vi "myRIO_BRig_RT__Case_Exp_State_Cue1__v2.vi"(6 "input_LC":bool, 7 "I_lick":bool, 8 "input_LC_led":bool, 10 "input_state":T1, 11 "input_dataCurrent":u16[](array[numeric])) -> (0 "output_trigger_laser_led":bool, 2 "output_state":T1, 3 "output_dataCurrent":u16[](array[numeric]), 4 "output_trigger_laser":bool)   [LabVIEW 2014]
uses:
  myRIO_BRig_RT__Case_Exp_stateList.ctl
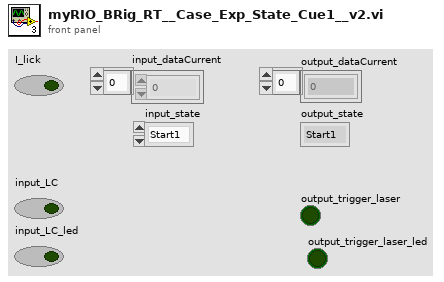
[diagram p1: front panel]
types:
  T1 = typedef "myRIO_BRig_RT__Case_Exp_stateList.ctl" = enum16{"Start1", "Start2", "Start3", "saveSettings1", "saveSettings2", "saveSettings3", "saveSettings4_LC_l1_ENL", "saveSettings4_LC_l2_ENL", "saveSettings5_LC_l1_Cue", "saveSettings5_LC_l2_Cue", "saveSettings6_LC_l1_Other", "SaveSettings6_LC_l2_Other", "setSettings_Audio", "setSettings_Laser", "initBlock_pre", "initBlock", "initBlock2", "initBlock_post", "initTrial_pre", "initTrial", "initTrial2", "initTrial3", "initTrial4", "initTrial_LC_ENL1", "initTrial_LC_Cue1", "initTrial_LC_Sel", "initTrial_post", "ENL1_pre", "ENL1", "ENL1_post", "ENL1Penalty_pre", "ENL1Penalty", "ENL2_pre", "ENL2", "ENL2Penalty_pre", "ENL2Penalty", "Cue1_pre", "Cue1", "Cue1_post", "Cue1Penalty_pre", "Cue1Penalty", "Cue2_pre", "Cue2", "Cue2Penalty_pre", "Cue2Penalty", "Selection_pre", "Selection", "Select_post", "SelectReward_pre", "SelectReward", "SelectRewardPost_pre", "SelectRewardPost", "SelectWrong_pre", "SelectWrong", "SelectWrong_post", "SelectTimeout_pre", "SelectTimeout", "SelectTimeout_post", "endTrial_pre", "endTrial1", "endTrial2", "endTrial3", "endTrial_post", "endBlock_pre", "endBlock", "endBlock_post", "endExp", "commConnect", "commUpload_pre", "commUpload_dataBlock", "commUpload_dataCurrent", "commUpload_dataExp", "commUpload_dataLC", "commUpload_dataTrial", "commUpload_post", "saveData_pre", "saveData_dataBlock", "saveData_dataCurrent", "saveData_dataExp", "saveData_dataLC", "saveData_dataTrial", "saveData_post", "empty_endBlock1", "empty_endBlock2", "empty_endTrial1", "empty_endTrial2", "empty_endTrial3", "empty_endTrial4", "empty_endTrial5", "dummyState", "dummyState_endBlock"}
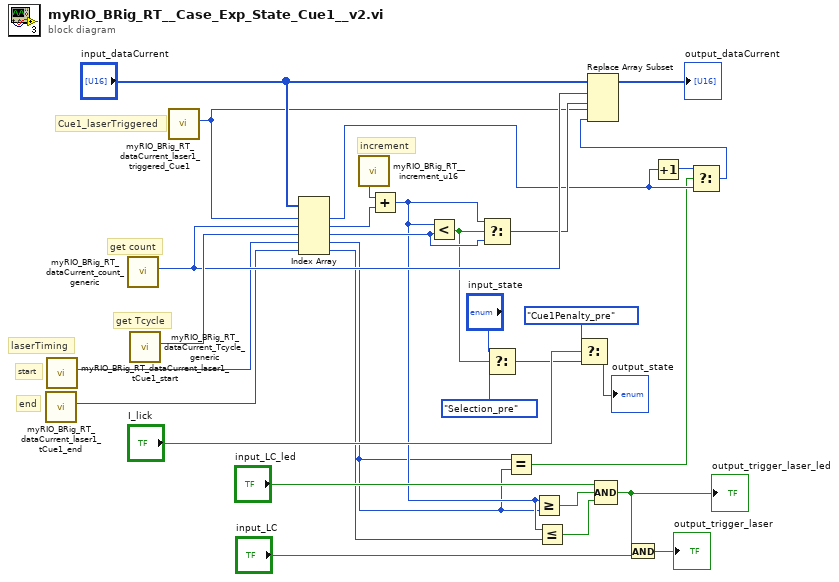
[diagram p0: block diagram]
diagram:
  # "Cue1_laserTriggered"
  # "end"
  # "start"
  # "laserTiming"
  # "increment"
  # "get Tcycle"
  # "get count"
  n1 = call "myRIO_BRig_RT_dataCurrent_laser1_tCue1_end.vi"() -> ("output_laser1_tCue1_end"=w9:i32)  [unwired: 11 in]
  n2 = call "myRIO_BRig_RT_dataCurrent_laser1_tCue1_start.vi"() -> ("output_laser1_tCue1_start"=w10:i32)  [unwired: 11 in]
  n3 = call "myRIO_BRig_RT_dataCurrent_count_generic.vi"() -> ("output_count_generic"=w28:i32)  [unwired: 11 in]
  n4 = call "myRIO_BRig_RT_dataCurrent_Tcycle_generic.vi"() -> ("output_Tcycle_generic"=w29:i32)  [unwired: 11 in]
  n5 = call "myRIO_BRig_RT_dataCurrent_laser1_triggered_Cue1.vi"() -> ("output_laser1_triggered_Cue1"=w8:i32)  [unwired: 11 in]
  n6 = Index Array(array="input_dataCurrent", index #1=w8, index #2=w28, index #3=w29, index #4=w10, index #5=w9) -> (element #1=w6:u16, element #2=w3:u16, element #3=w27:u16, element #4=w1:u16, element #5=w13:u16)
  n7 = call "myRIO_BRig_RT__increment_u16.vi"() -> ("output_increment__u16"=w22:u16)  [unwired: 11 in]
  n8 = Add(x=w22, y=w3) -> (x+y=w4:u16)
  n9 = Less?(x=w4, y=w27) -> (x < y?=w24:bool)
  n10 = Select(t=w4, s=w24, f=w27) -> (s? t:f=w26:u16)
  n11 = Select(t="input_state", s=w24, f=myRIO_BRig_RT__Case_Exp_stateList."Selection_pre" ("Enum")) -> (s? t:f=w23:T1)
  n12 = Equal?(x=w1, y=w1) -> (x = y?=w2:bool)
  n13 = Greater Or Equal?(x=w4, y=w1) -> (x >= y?=w20:bool)
  n14 = Less Or Equal?(x=w4, y=w13) -> (x <= y?=w21:bool)
  n15 = Select(t=myRIO_BRig_RT__Case_Exp_stateList."Cue1Penalty_pre" ("Enum"), s="I_lick", f=w23) -> (s? t:f=→"output_state":T1)
  n16 = Compound Arithmetic op=AND("input_LC_led", w20, w21) -> (w5:bool)
  "output_trigger_laser_led" <- w5
  n17 = And(x=w5, y="input_LC") -> (x .and. y?=→"output_trigger_laser":bool)
  n18 = Increment(x=w6) -> (x+1=w7:u16)
  n19 = Select(t=w7, s=w2, f=w6) -> (s? t:f=w11:u16)
  n20 = Replace Array Subset(array="input_dataCurrent", new element #1=w26, index #1=w28, new element #2=w11, index #2=w8) -> (→"output_dataCurrent":u16[])
